vi "resonanceAnalyzer.vi"() -> ()   [LabVIEW 2015]
uses:
  <vilib>/imath/engines/lvmath2/RunTimeEngine/Managers/WorkSpace/UID Generator.vi
  <vilib>/imath/engines/lvmath2/RunTimeEngine/RangeToken/NIMS_Range.vi
  <instcachedir>/0/NIMS_Range_D919CC09935940E88F755EC1C6F49AC1.lvgen/NIMS_Range_D919CC09935940E88F755EC1C6F49AC1_000.vi
  <vilib>/imath/engines/lvmath2/RunTimeEngine/RunTimeType/NIMS_RunTimeType_From StrictType (excl LVString).vi
  <instcachedir>/0/NIMS_RunTimeType_From StrictType (excl LVString)_EB1C38A9BC5048DA9ABDA8F781E54D21.lvgen/NIMS_RunTimeType_From StrictType (excl LVString)_EB1C38A9BC5048DA9ABDA8F781E54D21_000.vi
  <vilib>/imathl/engines/lvmath/Functions/Error Handling/Create Error.vi
  <vilib>/imath/engines/lvmath2/RunTimeEngine/LocalVariableDefStatement/MC_LocalVariableDefStatement_Display.vi
  <vilib>/imath/engines/lvmath2/RunTimeEngine/BuiltInFunctions/length/NIMS_length(GV).vi
  <instcachedir>/0/NIMS_length(GV)_08A3D13377FD4E4B96F5795FBF3698FA.lvgen/NIMS_length(GV)_08A3D13377FD4E4B96F5795FBF3698FA_000.vi
  <vilib>/imath/engines/lvmath2/RunTimeEngine/Managers/SymbolTable/Clear UID.vi
  <vilib>/imath/engines/lvmath2/RunTimeEngine/NodeEndStatement/NIMS_NodeEndStatement_Output.vi
  <instcachedir>/0/NIMS_NodeEndStatement_Output_53EC0D466D134D7ABD903AC30B43404B.lvgen/NIMS_NodeEndStatement_Output_53EC0D466D134D7ABD903AC30B43404B_013.vi
  <instcachedir>/0/NIMS_NodeEndStatement_Output_53EC0D466D134D7ABD903AC30B43404B.lvgen/NIMS_NodeEndStatement_Output_53EC0D466D134D7ABD903AC30B43404B_005.vi
  <vilib>/imath/engines/lvmath2/RunTimeEngine/ErrorHandling/NIMS_Finalize Error.vi
  <vilib>/addons/Time Series Analysis/Utilities.llb/TSA Normal Distribution (Waveform).vi
  <vilib>/imath/engines/lvmath2/RunTimeEngine/ArithmeticOperatorToken/NIMS_ArithmeticOperator_plus.vi
  <instcachedir>/0/NIMS_ArithmeticOperator_plus_A4F2756F5ADB4A0090E0DBD7C10701C8.lvgen/NIMS_ArithmeticOperator_plus_A4F2756F5ADB4A0090E0DBD7C10701C8_004.vi
  <vilib>/imath/engines/lvmath2/RunTimeEngine/ArithmeticOperatorToken/NIMS_ArithmeticOperator_rightdiv.vi
  <instcachedir>/0/NIMS_ArithmeticOperator_rightdiv_E8FF7CD3D5774FA6AA728C3F0517CAD4.lvgen/NIMS_ArithmeticOperator_rightdiv_E8FF7CD3D5774FA6AA728C3F0517CAD4_000.vi
  <vilib>/imath/engines/lvmath2/RunTimeEngine/ErrorHandling/NIMS_Create Error From Enums.vi
  <vilib>/Utility/file.llb/Read Delimited Spreadsheet (DBL).vi
  <vilib>/imath/engines/lvmath2/RunTimeEngine/BuiltInFunctions/max/1 input/NIMS_max(RV).vi
  <instcachedir>/0/NIMS_max(RV)_237633DB1D604D5BA7001287DF3C7957.lvgen/NIMS_max(RV)_237633DB1D604D5BA7001287DF3C7957_000.vi
  <instcachedir>/0/NIMS_NodeEndStatement_Output_53EC0D466D134D7ABD903AC30B43404B.lvgen/NIMS_NodeEndStatement_Output_53EC0D466D134D7ABD903AC30B43404B_001.vi
  <vilib>/imath/engines/lvmath2/RunTimeEngine/Managers/SymbolTable/NIMS_WorkSpace.lvlib
  <vilib>/addons/_Advanced Signal Processing/NI_AdvSigProcTSA.lvlib
panel:
  out "Results":cluster{"w0":dbl, "Q":dbl, "amp":dbl}={"w0"=600.1256549934647, "Q"=5.096176964863202, "amp"=0.8232181396050281}
  out "Data Graph":cluster{"all rows":dbl[], "Array":dbl[]}[](graph)
  in  "Data Control":enum32{"Simulation", "Experiment"}(tab)=enum."Experiment"
  in  "Input Parameters":T1={"Start Frequency"=400.0, "End Frequency"=800.0, "df"=5.0, "Noise Level"=0.05, "Resonant Frequency"=600.0, "Q"=5.0}
  in  "Filename":path=path "U:/PHYS 434/Homework 5/resData"
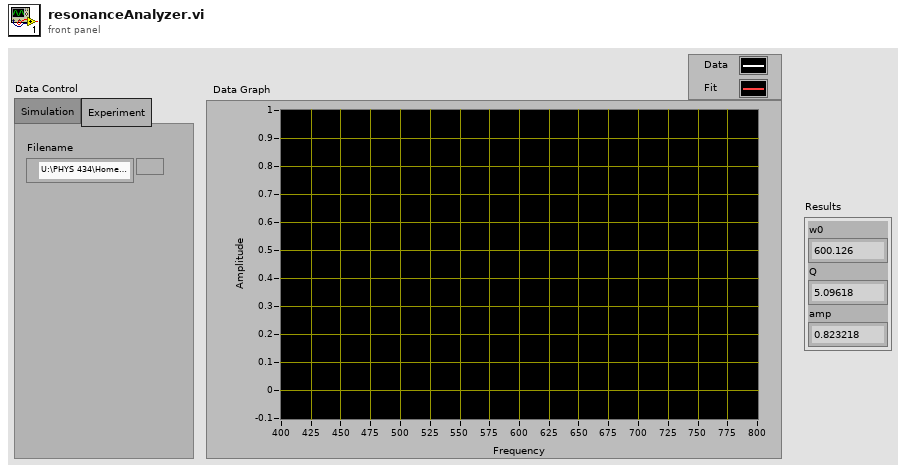
[diagram p1: front panel]
types:
  T1 = cluster{"Start Frequency":dbl, "End Frequency":dbl, "df":dbl, "Noise Level":dbl, "Resonant Frequency":dbl, "Q":dbl}
  T2 = cluster{"Array[0]":dbl, "Array[1]":dbl, "Array[2]":dbl, "Array[3]":dbl, "Array[4]":dbl, "Array[5]":dbl, "Array[6]":dbl, "Array[7]":dbl, "Array[8]":dbl}
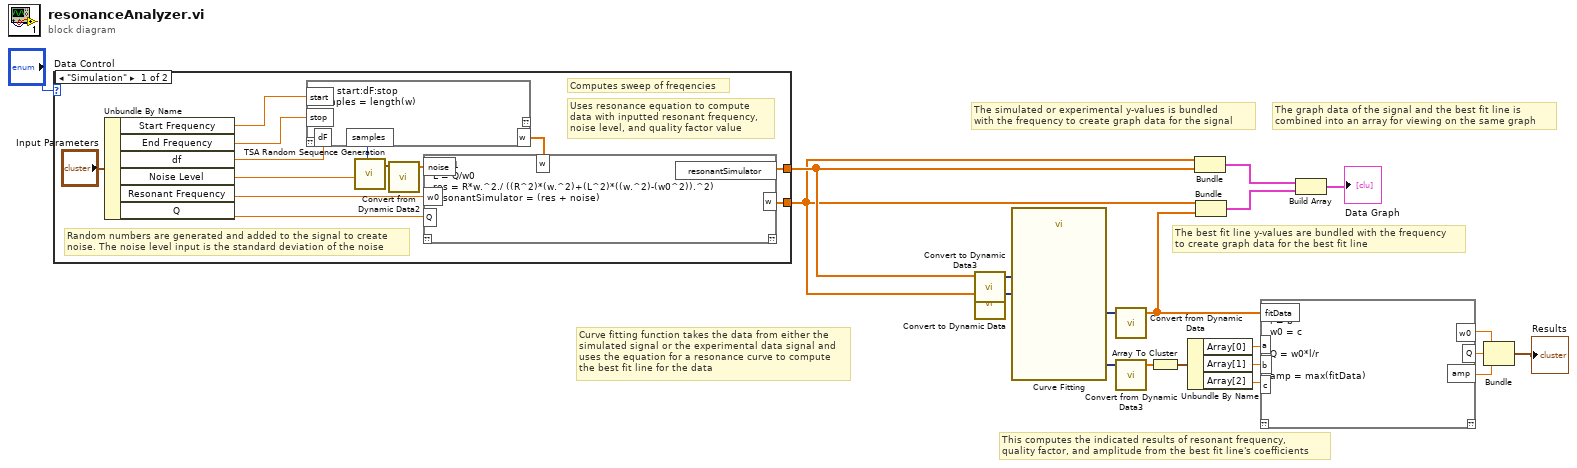
[diagram p0: block diagram]
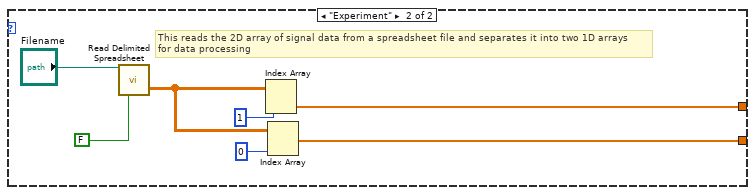
[diagram p2: hidden frame]
diagram:
  # "This computes the indicated results of resonant frequency, \nquality factor, and amplitude from the best fit line's coefficients"
  # "Curve fitting function takes the data from either the \nsimulated signal or the experimental data signal and\nuses the equation for a resonance curve to compute\nthe best fit line for the data"
  # "The graph data of the signal and the best fit line is \ncombined into an array for viewing on the same graph"
  # "The best fit line y-values are bundled with the frequency\nto create graph data for the best fit line"
  # "The simulated or experimental y-values is bundled \nwith the frequency to create graph data for the signal"
  n1 = case shown="\"Simulation\"" "Data Control" {
    tunnel: [w24 w235] -> w1
    tunnel: [w23 w236] -> w6
    frame "Simulation" {
      # "Random numbers are generated and added to the signal to create\nnoise. The noise level input is the standard deviation of the noise"
      # "Uses resonance equation to compute\ndata with inputted resonant frequency,\nnoise level, and quality factor value"
      # "Computes sweep of freqencies"
      n2 = Unbundle By Name("Input Parameters") -> ("Start Frequency"=w26:dbl, "End Frequency"=w21:dbl, "df"=w27:dbl, "Noise Level"=w22:dbl, "Resonant Frequency"=w30:dbl, "Q"=w31:dbl)
      n3 = mathscript code="w = start:dF:stop\nsamples = length(w)"("start"=w26, "stop"=w21, "dF"=w27) -> ("w"=w25:dbl[], "samples"=w29:i32)  [unwired: 1 in, 1 out]
      n4 = call-poly <vilib>:"TSA Random Sequence Generation.vi"("standard deviation"=w22, "samples"=w29) -> ("Xt"=w32:waveform(dbl))  [unwired: 8 in, 1 out]
      n5 = call "Convert from Dynamic Data2"("Dynamic Data Type"=w32) -> ("Array"=w33:dbl[])  [unwired: 3 in]
      n6 = mathscript code="R = 1\nL = Q/w0\nres = R*w.^2./ ((R^2)*(w.^2)+(L^2)*((w.^2)-(w0^2)).^2)\nresonantSimulator = (res + noise)"("w0"=w30, "Q"=w31, "w"=w25, "noise"=w33) -> ("resonantSimulator"=w23:dbl[], "w"=w24:dbl[])  [unwired: 1 in, 1 out]
    }
    frame "Experiment" {
      # "This reads the 2D array of signal data from a spreadsheet file and separates it into two 1D arrays\nfor data processing"
      n7 = call-poly <vilib>:"Read Delimited Spreadsheet.vi"("file path (dialog if empty)"="Filename", "transpose? (F)"=FALSE) -> ("all rows"=w238:dbl[][])  [unwired: 8 in, 5 out]
      n8 = Index Array(array=w238, index (col)=1 ("disabled index (col)")) -> (element=w236:dbl[])  [unwired: 1 in]
      n9 = Index Array(array=w238, index (col)=0 ("disabled index (col)")) -> (element=w235:dbl[])  [unwired: 1 in]
    }
  }
  n10 = call "Convert to Dynamic Data3"("Array"=w6) -> ("Dynamic Data Type"=w7:dynamicdata)  [unwired: 3 in]
  n11 = call "Convert to Dynamic Data"("Array"=w1) -> ("Dynamic Data Type"=w8:dynamicdata)  [unwired: 3 in]
  n12 = call "Curve Fitting"("Locations"=w8, "Signals"=w7) -> ("best fit"=w9:dynamicdata, "non-linear coefficients"=w10:dynamicdata)  [unwired: 5 in, 3 out]
  n13 = call "Convert from Dynamic Data"("Dynamic Data Type"=w9) -> ("Array"=w2:dbl[])  [unwired: 3 in]
  n14 = call "Convert from Dynamic Data3"("Dynamic Data Type"=w10) -> ("Array"=w11:dbl[])  [unwired: 3 in]
  n15 = Array To Cluster(array=w11) -> (cluster=w12:T2)
  n16 = Unbundle By Name(w12) -> ("Array[0]"=w13:dbl, "Array[1]"=w14:dbl, "Array[2]"=w15:dbl)
  n17 = Bundle("all rows"=w1, "all rows"=w6) -> (w5:cluster{"all rows":dbl[], "all rows":dbl[]})  [unwired: 1 in]
  n18 = Bundle("all rows"=w1, "Array"=w2) -> (w4:cluster{"all rows":dbl[], "Array":dbl[]})  [unwired: 1 in]
  n19 = mathscript code="r = a\nl = b\nw0 = c\n\nQ = w0*l/r\n\namp = max(fitData)"("a"=w13, "b"=w14, "c"=w15, "fitData"=w2) -> ("amp"=w18:dbl, "Q"=w16:dbl, "w0"=w17:dbl)  [unwired: 1 in, 1 out]
  n20 = Build Array(w5, w4) -> (→"Data Graph":cluster{"all rows":dbl[], "Array":dbl[]}[])
  n21 = Bundle("w0"=w17, "Q"=w16, "amp"=w18) -> (→"Results":cluster{"w0":dbl, "Q":dbl, "amp":dbl})  [unwired: 1 in]
